vi "pmu_Configuration Block CFG-3.vi"(5 "CFG-3 PMU location":T1, 7 "CFG-3 dynamci response factors [us]":T2, 9 "CFG-3 class":T3={"station name"="", "PMU ID"=0, "global PMU ID"=38528, "time base"=1, "nominal frequency"=enum."60 Hz", "reporting rate"=0, "phasor number"=0, "analog number"=0, "digital number"=0, "channel names"=[], "phasor scale first 4 bytes"=[], "phasor scale factors"=[], "phasor angle offsets [rad]"=[], "analog scale factors"=[], "analog magnitude offsets"=[], "digital units"=[], "data format"=15, "number of PMUs"=1} {"digital units" format="%.0x"}, 10 "performance class":enum8{"M Class", "P Class"}(ring), 11 "configuration change count":u16) -> (3 "data":u8[](array[numeric]))   [LabVIEW 2014, in "NI_EP_PMU.lvlib"]
doc: "This VI builds IEEE C37.118-2005 configuration message frame sent by the PMU."
uses:
  <vilib>/addons/Electrical Power/PMU/NI_EP_PMU.lvlib
  <vilib>/addons/Electrical Power/PMU/Common/Controls/pmu_CFG-3 Class.ctl
  <vilib>/addons/Electrical Power/PMU/Common/Controls/pmu_CFG-3 Dynamic Response Factors.ctl
  <vilib>/addons/Electrical Power/PMU/Common/Controls/pmu_CFG-3 PMU location.ctl
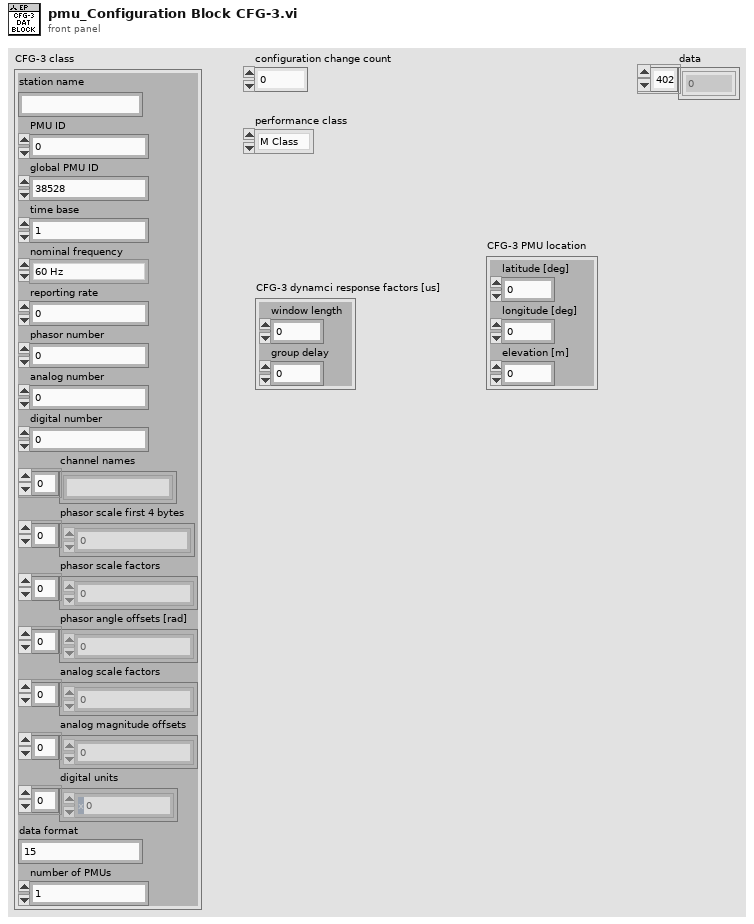
[diagram p1: front panel]
types:
  T1 = typedef "NI_EP_PMU.lvlib/pmu_CFG-3 PMU location.ctl" = cluster{"latitude [deg]":sgl, "longitude [deg]":sgl, "elevation [m]":sgl}
  T2 = typedef "NI_EP_PMU.lvlib/pmu_CFG-3 Dynamic Response Factors.ctl" = cluster{"window length":i32, "group delay":i32}
  T3 = typedef "NI_EP_PMU.lvlib/pmu_CFG-3 Class.ctl" = cluster{"station name":string, "PMU ID":u16, "global PMU ID":u64, "time base":u32, "nominal frequency":enum16{"50 Hz", "60 Hz"}, "reporting rate":i16, "phasor number":u16, "analog number":u16, "digital number":u16, "channel names":string[], "phasor scale first 4 bytes":u32[], "phasor scale factors":sgl[], "phasor angle offsets [rad]":sgl[], "analog scale factors":sgl[], "analog magnitude offsets":sgl[], "digital units":u32[], "data format":u16, "number of PMUs":u16}
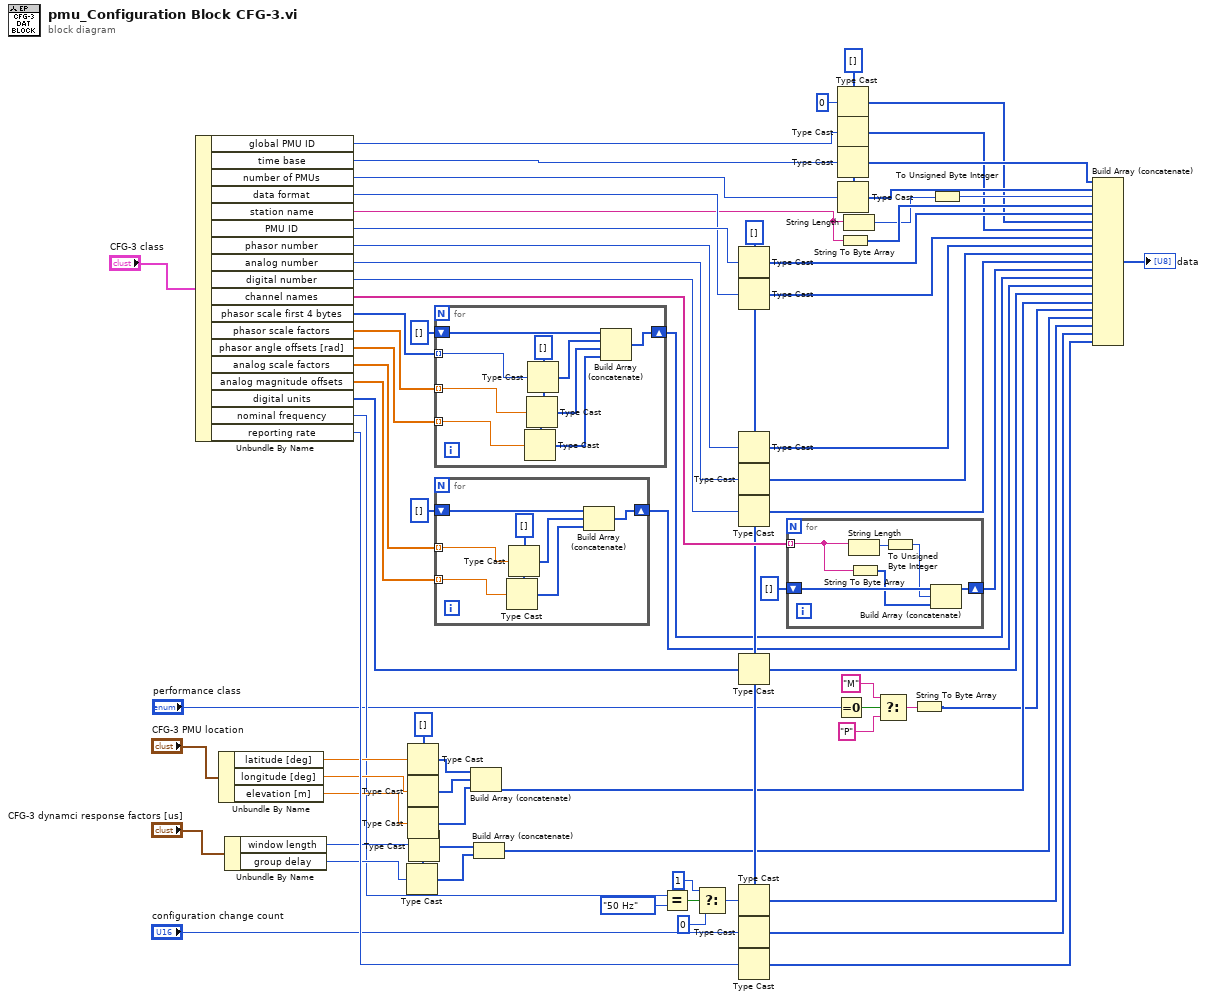
[diagram p0: block diagram]
diagram:
  w29 = u8[] [] ("appended array")
  w49 = u8[] [] ("appended array")
  w15 = u8[] [] ("appended array")
  n1 = Unbundle By Name("CFG-3 class") -> ("global PMU ID"=w14:u64, "time base"=w60:u32, "number of PMUs"=w59:u16, "data format"=w58:u16, "station name"=w21:string, "PMU ID"=w66:u16, "phasor number"=w65:u16, "analog number"=w64:u16, "digital number"=w63:u16, "channel names"=w72:string[], "phasor scale first 4 bytes"=w51:u32[], "phasor scale factors"=w9:sgl[], "phasor angle offsets [rad]"=w8:sgl[], "analog scale factors"=w7:sgl[], "analog magnitude offsets"=w6:sgl[], "digital units"=w70:u32[], "nominal frequency"=w17:enum16{"50 Hz", "60 Hz"}, "reporting rate"=w62:i16)
  n2 = Unbundle By Name("CFG-3 PMU location") -> ("latitude [deg]"=w45:sgl, "longitude [deg]"=w44:sgl, "elevation [m]"=w43:sgl)
  n3 = Unbundle By Name("CFG-3 dynamci response factors [us]") -> ("window length"=w28:i32, "group delay"=w27:i32)
  n4 = Type Cast(type=w29, x=w45) -> (*(type *) &x=w42:u8[])
  n5 = Type Cast(type=w29, x=w44) -> (*(type *) &x=w41:u8[])
  n6 = Type Cast(type=w29, x=w43) -> (*(type *) &x=w40:u8[])
  n7 = Type Cast(type=w29, x=w28) -> (*(type *) &x=w26:u8[])
  n8 = Type Cast(type=w26, x=w27) -> (*(type *) &x=w25:u8[])
  n9 = for {
    tunnel: w51 -> [w75] mode=indexing
    shift-right: [w81] -> w31
    shift-left: u8[] [] -> [w80]
    tunnel: w9 -> [w74] mode=indexing
    tunnel: w8 -> [w73] mode=indexing
    w79 = u8[] [] ("appended array")
    n10 = Type Cast(type=w79, x=w74) -> (*(type *) &x=w77:u8[])
    n11 = Type Cast(type=w77, x=w73) -> (*(type *) &x=w76:u8[])
    n12 = Type Cast(type=w79, x=w75) -> (*(type *) &x=w78:u8[])
    n13 = Build Array (concatenate)(w80, w78, w77, w76) -> (w81:u8[])
  }
  n14 = for {
    shift-right: [w88] -> w30
    shift-left: u8[] [] -> [w87]
    tunnel: w7 -> [w83] mode=indexing
    tunnel: w6 -> [w82] mode=indexing
    n15 = Type Cast(type=u8[] [] ("appended array"), x=w83) -> (*(type *) &x=w85:u8[])
    n16 = Type Cast(type=w85, x=w82) -> (*(type *) &x=w84:u8[])
    n17 = Build Array (concatenate)(w87, w85, w84) -> (w88:u8[])
  }
  n18 = Build Array (concatenate)(w42, w41, w40) -> (w18:u8[])
  n19 = Build Array (concatenate)(w26, w25) -> (w24:u8[])
  n20 = Equal?(x=w17, y=enum16{"50 Hz", "60 Hz"}."50 Hz" ("nominal frequency")) -> (x = y?=w57:bool)
  n21 = Select(t=u16 1, s=w57, f=u16 0) -> (s? t:f=w53:u16)
  n22 = Type Cast(type=w49, x=w66) -> (*(type *) &x=w38:u8[])
  n23 = Type Cast(type=w49, x=w58) -> (*(type *) &x=w37:u8[])
  n24 = Type Cast(type=w49, x=w65) -> (*(type *) &x=w36:u8[])
  n25 = Type Cast(type=w49, x=w64) -> (*(type *) &x=w35:u8[])
  n26 = Type Cast(type=w49, x=w63) -> (*(type *) &x=w34:u8[])
  n27 = Type Cast(type=w49, x=w70) -> (*(type *) &x=w32:u8[])
  n28 = Type Cast(type=w49, x=w53) -> (*(type *) &x=w69:u8[])
  n29 = Type Cast(type=w49, x="configuration change count") -> (*(type *) &x=w68:u8[])
  n30 = Type Cast(type=w49, x=w62) -> (*(type *) &x=w67:u8[])
  n31 = for {
    shift-right: [w93] -> w33
    shift-left: u8[] [] -> [w94]
    tunnel: w72 -> [w92] mode=indexing
    n32 = String Length(string=w92) -> (length=w90:i32)
    n33 = String To Byte Array(string=w92) -> (unsigned byte array=w91:u8[])
    n34 = To Unsigned Byte Integer(number=w90) -> (unsigned 8bit integer=w89:u8)
    n35 = Build Array (concatenate)(w94, w89, w91) -> (w93:u8[])
  }
  n36 = Equal To 0?(x="performance class") -> (x = 0?=w5:bool)
  n37 = Type Cast(type=w15, x=u64 0) -> (*(type *) &x=w13:u8[])
  n38 = Type Cast(type=w15, x=w14) -> (*(type *) &x=w12:u8[])
  n39 = Type Cast(type=w15, x=w60) -> (*(type *) &x=w16:u8[])
  n40 = Type Cast(type=w15, x=w59) -> (*(type *) &x=w39:u8[])
  n41 = String To Byte Array(string=w21) -> (unsigned byte array=w22:u8[])
  n42 = String Length(string=w21) -> (length=w20:i32)
  n43 = Select(t="M", s=w5, f="P") -> (s? t:f=w2:string)
  n44 = String To Byte Array(string=w2) -> (unsigned byte array=w1:u8[])
  n45 = To Unsigned Byte Integer(number=w20) -> (unsigned 8bit integer=w19:u8)
  n46 = Build Array (concatenate)(w16, w39, w19, w22, w38, w13, w12, w37, w36, w35, w34, w33, w31, w30, w32, w18, w1, w24, w69, w68, w67) -> (→"data":u8[])
